vi "Stimulation.vi"(8 "Error in":errorcluster, 10 "Device parameters":T1={"Stimulation channel"="Dev1/ao0", "Stimulation sample rate"=10000.0} {"Stimulation sample rate" min=10.0 max=10000.0}) -> ()   [LabVIEW 2014]
uses:
  <vilib>/DAQmx/write.llb/DAQmx Write (Analog 1D DBL 1Chan NSamp).vi
  <vilib>/DAQmx/create/channels.llb/DAQmx Create Channel (AO-Voltage-Basic).vi
  <vilib>/DAQmx/configure/timing.llb/DAQmx Timing (Sample Clock).vi
  <vilib>/DAQmx/configure/trigger.llb/DAQmx Start Trigger (Digital Edge).vi
  <vilib>/DAQmx/miscellaneous.llb/DAQmx Fill In Error Info.vi
panel:
  in  "Baseline":dbl
  in  "OFF time":dbl=60.0
  in  "ON time":dbl=10.0
  in  "Pulse width":dbl=0.0005
  in  "Repetitions":dbl=15.0
  in  "Stim Freq":dbl=1.0 format="%#_13g"
  in  "Triggered?":bool
  # "STIMULATOR"
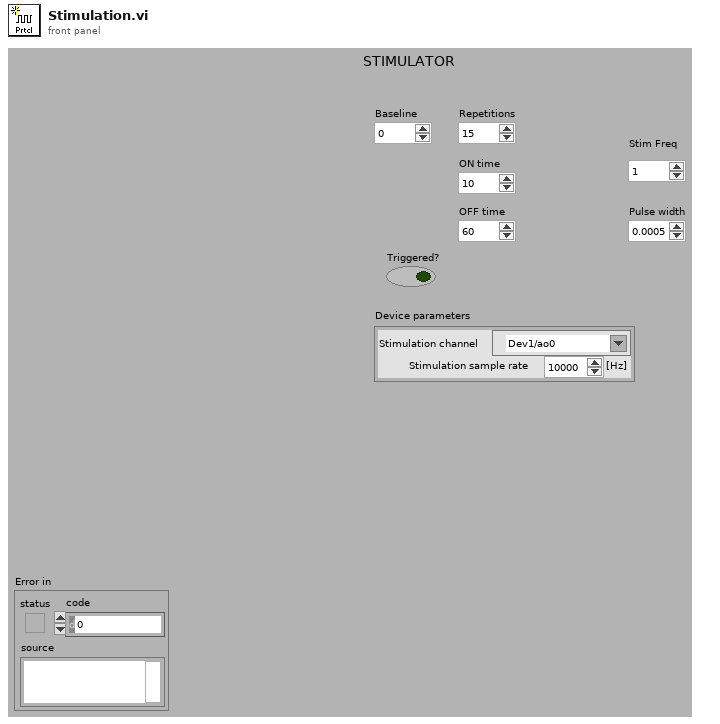
[diagram p1: front panel]
types:
  T1 = cluster{"Stimulation channel":tag, "Stimulation sample rate":dbl}
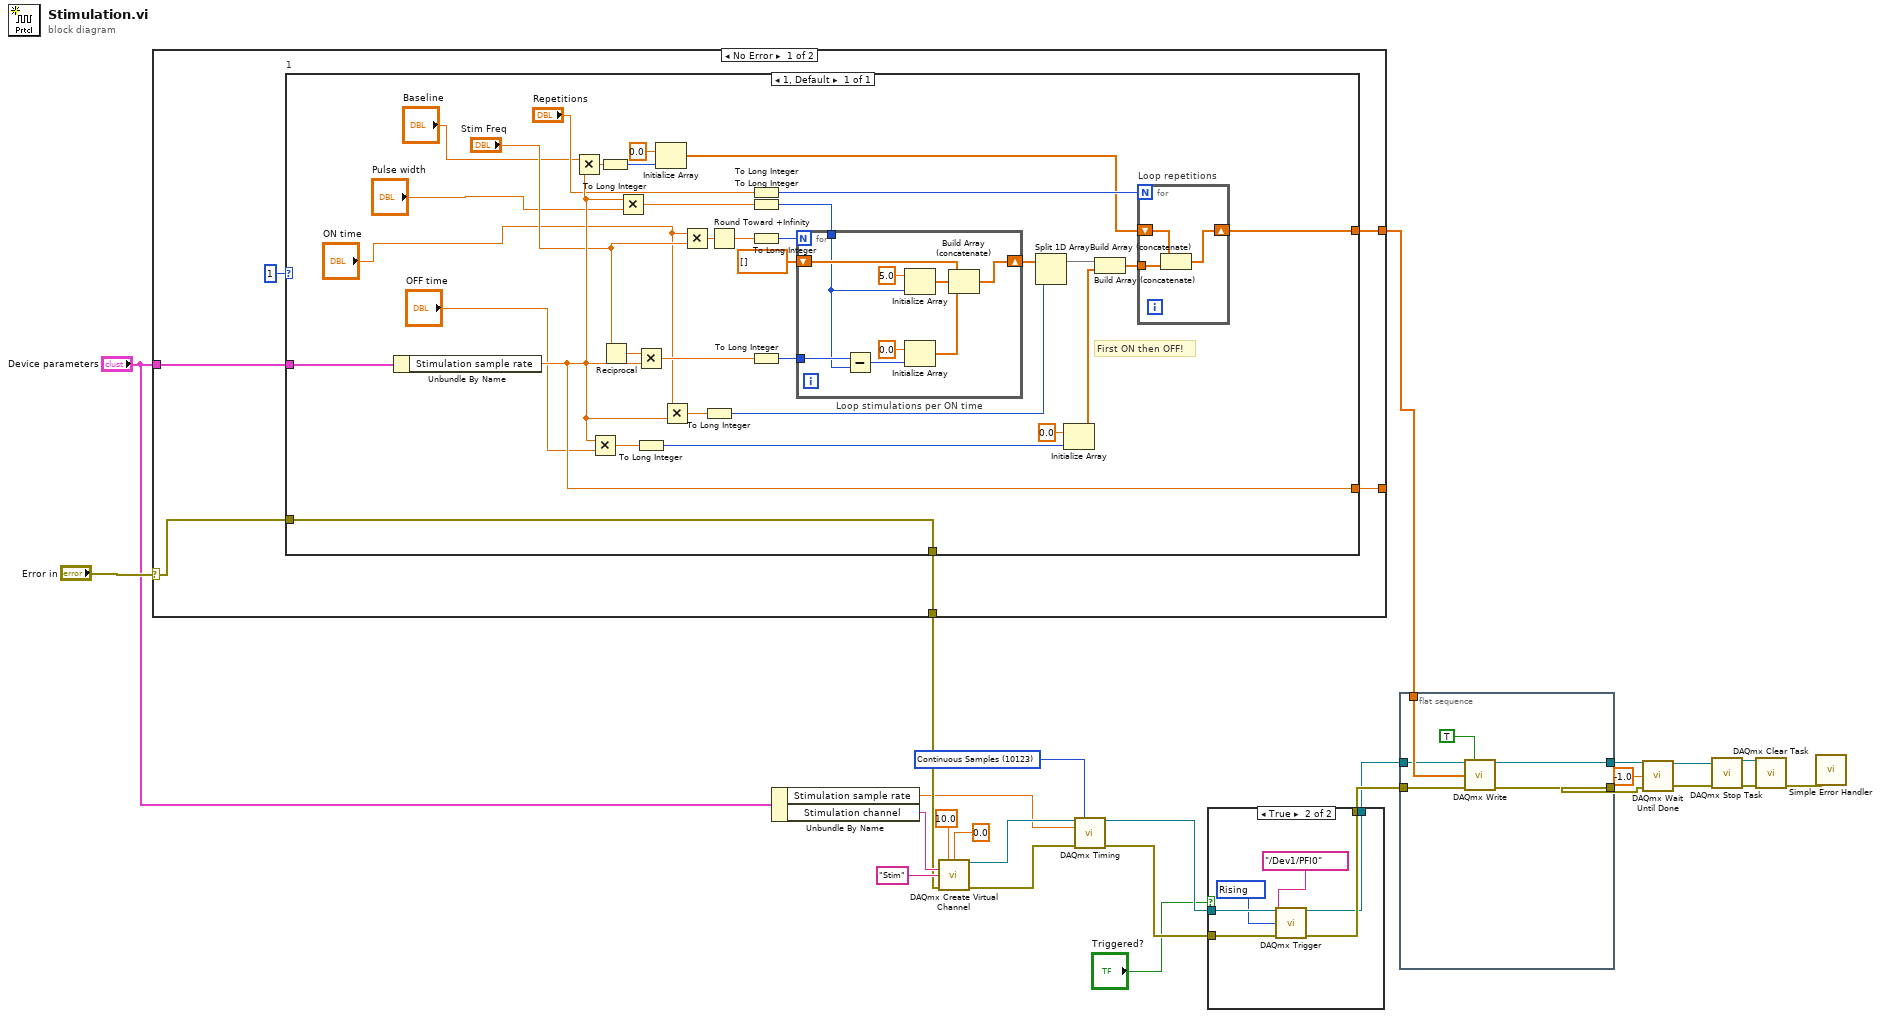
[diagram p0: block diagram]
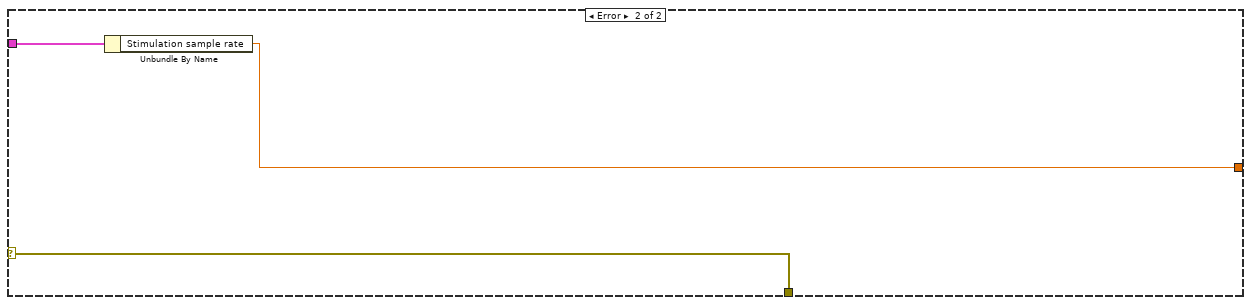
[diagram p3: hidden frame]
diagram:
  w15 = 10123 items=["Finite Samples"=10178, "Continuous Samples"=10123, "Hardware Timed Single Point"=12522] ("sample mode")
  n1 = case shown="No Error" "Error in" {
    selector: "Error in" -> [w30 w79]
    tunnel: "Device parameters" -> [w31 w78]
    tunnel: [w27 _] -> w14
    tunnel: [w29 w79] -> w19
    tunnel: [w28 w77] -> _
    frame No Error {
      n2 = case "1" shown="1, Default" 1 {
        tunnel: w31 -> [w61]
        tunnel: w30 -> [w40]
        tunnel: [w40] -> w29
        tunnel: [w39] -> w28
        tunnel: [w33] -> w27
        frame 1, Default {
          # "First ON then OFF!"
          n3 = Unbundle By Name(w61) -> ("Stimulation sample rate"=w39:dbl)
          n4 = Multiply(x="Baseline", y=w39) -> (x*y=w48:dbl)
          n5 = Multiply(x=w39, y="OFF time") -> (x*y=w53:dbl)
          n6 = To Long Integer(number=w48) -> (32bit integer=w47:i32)
          n7 = Reciprocal(x="Stim Freq") -> (1/x=w60:dbl)
          n8 = Multiply(x=w39, y="Pulse width") -> (x*y=w44:dbl)
          n9 = Multiply(x=w60, y=w39) -> (x*y=w46:dbl)
          n10 = To Long Integer(number=w53) -> (32bit integer=w52:i32)
          n11 = Initialize Array(0.0 ("element"), w47) -> (w49:dbl[])
          n12 = Multiply(x="ON time", y=w39) -> (x*y=w59:dbl)
          n13 = Multiply(x="ON time", y="Stim Freq") -> (x*y=w63:dbl)
          n14 = To Long Integer(number=w59) -> (32bit integer=w55:i32)
          n15 = Round Toward +Infinity(x=w63) -> (ceil(x): smallest int >= x=w62:dbl)
          n16 = To Long Integer(number="Repetitions") -> (32bit integer=w51:i32)
          n17 = To Long Integer(number=w44) -> (32bit integer=w43:i32)
          n18 = To Long Integer(number=w62) -> (32bit integer=w57:i32)
          n19 = To Long Integer(number=w46) -> (32bit integer=w45:i32)
          n20 = for "Loop stimulations per ON time" {
            N: w57 -> [_]
            tunnel: w45 -> [w75]
            tunnel: w43 -> [w69]
            shift-right: [w70] -> w56
            shift-left: dbl[] [] -> [w71]
            n21 = Subtract(x=w75, y=w69) -> (x-y=w68:i32)
            n22 = Initialize Array(5.0 ("element"), w69) -> (w73:dbl[])
            n23 = Initialize Array(0.0 ("element"), w68) -> (w72:dbl[])
            n24 = Build Array (concatenate)(w71, w73, w72) -> (w70:dbl[])
          }
          n25 = Split 1D Array(array=w56, index=w55) -> (first subarray=w41:dbl[])  [unwired: 1 out]
          n26 = Initialize Array(0.0 ("element"), w52) -> (w42:dbl[])
          n27 = Build Array (concatenate)(w41, w42) -> (w50:dbl[])
          n28 = for "Loop repetitions" {
            N: w51 -> [_]
            shift-right: [w65] -> w33
            shift-left: w49 -> [w67]
            tunnel: w50 -> [w66]
            n29 = Build Array (concatenate)(w67, w66) -> (w65:dbl[])
          }
        }
      }
    }
    frame Error {
      n30 = Unbundle By Name(w78) -> ("Stimulation sample rate"=w77:dbl)
    }
  }
  n31 = Unbundle By Name("Device parameters") -> ("Stimulation sample rate"=w16:dbl, "Stimulation channel"=w24:tag)
  n32 = call-poly <vilib>:"DAQmx Create Virtual Channel.vi"("maximum value"=10.0, "minimum value"=0.0, "physical channels"=w24, "name to assign"="Stim", "error in"=w19) -> ("task out"=w17:refnum<k21>, "error out"=w18:errorcluster)  [unwired: 9 in]
  n33 = call-poly <vilib>:"DAQmx Timing.vi"("task/channels in"=w17, "sample mode"=w15, "rate"=w16, "error in"=w18) -> ("task out"=w3:refnum<k21>, "error out"=w5:errorcluster)  [unwired: 10 in]
  n34 = case shown="True" "Triggered?" {
    tunnel: w5 -> [w80 w87]
    tunnel: [w80 w86] -> w4
    tunnel: w3 -> [w81 w85]
    tunnel: [w81 w84] -> w2
    frame False {
    }
    frame True {
      w82 = 10280 items=["Rising"=10280, "Falling"=10171] ("edge")
      n35 = call-poly <vilib>:"DAQmx Trigger.vi"("task/channels in"=w85, "source"=tag "/Dev1/PFI0", "edge"=w82, "error in"=w87) -> ("task out"=w84:refnum<k21>, "error out"=w86:errorcluster)  [unwired: 10 in]
    }
  }
  n36 = flat-sequence {
    tunnel: w14 -> [w92]
    tunnel: [w91] -> w7
    tunnel: [w90] -> w6
    tunnel: w4 -> [w89]
    tunnel: w2 -> [w88]
    frame #0 {
      n37 = call-poly <vilib>:"DAQmx Write.vi"("task/channels in"=w88, "auto start"=TRUE, "data"=w92, "error in"=w89) -> ("task out"=w91:refnum<k21>, "error out"=w90:errorcluster)  [unwired: 9 in, 1 out]
    }
  }
  n38 = call <vilib>:"DAQmx Wait Until Done.vi"("task/channels in"=w7, "timeout (sec)"=-1.0, "error in"=w6) -> ("task out"=w10:refnum<k21>, "error out"=w9:errorcluster)  [unwired: 11 in]
  n39 = call <vilib>:"DAQmx Stop Task.vi"("task/channels in"=w10, "error in"=w9) -> ("task out"=w13:refnum<k21>, "error out"=w12:errorcluster)  [unwired: 12 in]
  n40 = call <vilib>:"DAQmx Clear Task.vi"("task in"=w13, "error in"=w12) -> ("error out"=w11:errorcluster)  [unwired: 13 in]
  n41 = call <vilib>:"Simple Error Handler.vi"("error in (no error)"=w11) -> ()  [unwired: 4 in, 5 out]
